vi "GaugeConv.vi"(2 "mbar?":bool, 3 "Pirani?":bool, 4 "V-To-P?":bool, 5 "Index":i32[](array[numeric]), 6 "Voltage":u32[](array[numeric]), 7 "Press":dbl[](array[numeric]) format="%.2f") -> (0 "Voltage out":u32[](array[numeric]), 1 "Press out":dbl[](array[numeric]) format="%.4e")   [LabVIEW 2011]
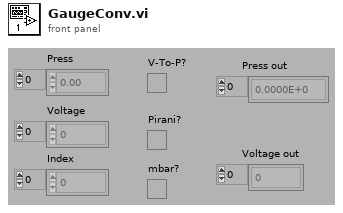
[diagram p1: front panel]
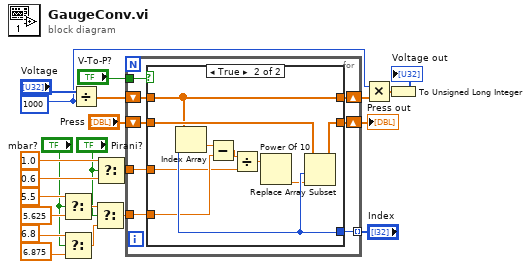
[diagram p0: block diagram]
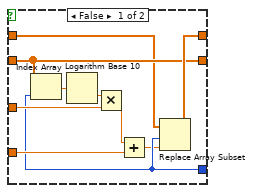
[diagram p2: hidden frame]
diagram:
  w1 = 1000
  n1 = Select(t=5.5, s="mbar?", f=5.625) -> (s? t:f=w15:dbl)
  n2 = Select(t=6.8, s="mbar?", f=6.875) -> (s? t:f=w13:dbl)
  n3 = Divide(x="Voltage", y=w1) -> (x/y=w6:dbl[])
  n4 = Select(t=w15, s="Pirani?", f=w13) -> (s? t:f=w12:dbl)
  n5 = Select(t=1.0, s="Pirani?", f=0.6) -> (s? t:f=w10:dbl)
  n6 = for {
    tunnel: "V-To-P?" -> [w23]
    tunnel: w12 -> [w30]
    tunnel: "Index" -> [w29] mode=indexing
    tunnel: w10 -> [w28]
    shift-right: [w26] -> w8
    shift-left: "Press" -> [w27]
    shift-right: [w24] -> w5
    shift-left: w6 -> [w25]
    n7 = case shown="True" w23 {
      tunnel: w30 -> [w40 w45]
      tunnel: w29 -> [w35 w50]
      tunnel: w28 -> [w38 w42]
      tunnel: [w34 w46] -> w24
      tunnel: w27 -> [w33 w48]
      tunnel: [w33 w47] -> w26
      tunnel: w25 -> [w32 w46]
      frame False {
        n8 = Index Array(array=w33, index=w35) -> (element=w39:dbl)
        n9 = Logarithm Base 10(1:w39) -> (0:w37:dbl)
        n10 = Multiply(x=w37, y=w38) -> (x*y=w36:dbl)
        n11 = Add(x=w36, y=w40) -> (x+y=w31:dbl)
        n12 = Replace Array Subset(array=w32, new element=w31, index=w35) -> (w34:dbl[])
      }
      frame True {
        n13 = Index Array(array=w46, index=w50) -> (element=w44:dbl)
        n14 = Subtract(x=w44, y=w45) -> (x-y=w43:dbl)
        n15 = Divide(x=w43, y=w42) -> (x/y=w41:dbl)
        n16 = Power Of 10(x=w41) -> (10^x=w49:dbl)
        n17 = Replace Array Subset(array=w48, new element=w49, index=w50) -> (w47:dbl[])
      }
    }
  }
  "Press out" <- w8
  n18 = Multiply(x=w1, y=w5) -> (x*y=w4:dbl[])
  n19 = To Unsigned Long Integer(number=w4) -> (unsigned 32bit integer=→"Voltage out":u32[])
